vi "Build Array.vi"(8 "Msg ID":u16, 9 "Total no of Bytes":u16, 11 "Array":u8[](array[numeric])) -> (2 "Array Packets":u8[][](array[numeric]))   [LabVIEW 2020]
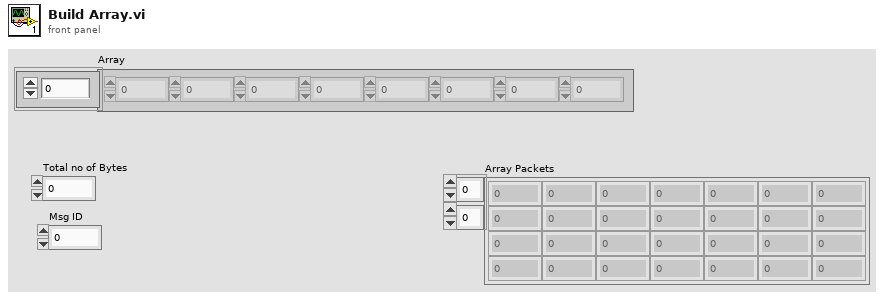
[diagram p1: front panel]
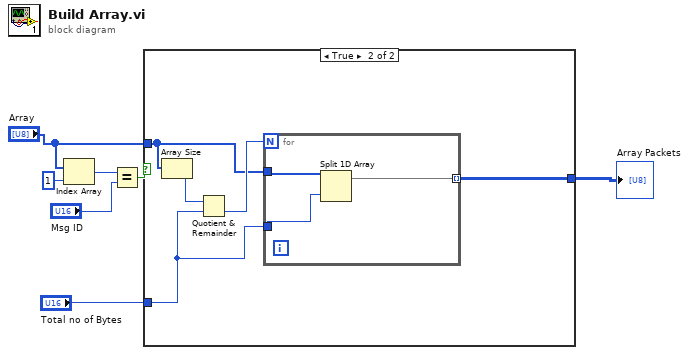
[diagram p0: block diagram]
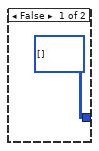
[diagram p2: hidden frame]
diagram:
  n1 = Index Array(array="Array", index=1) -> (element=w3:u8)
  n2 = Equal?(x=w3, y="Msg ID") -> (x = y?=w4:bool)
  n3 = case shown="True" w4 {
    tunnel: "Array" -> [_ w11]
    tunnel: "Total no of Bytes" -> [_ w10]
    tunnel: [u8[][] [] w9] -> w1
    frame False {
    }
    frame True {
      n4 = Array Size(array=w11) -> (size(s)=w13:i32)
      n5 = Quotient & Remainder(x=w13, y=w10) -> (floor(x/y)=w12:i32)  [unwired: 1 out]
      n6 = for {
        N: w12 -> [_]
        tunnel: w11 -> [w16]
        tunnel: w10 -> [w14]
        tunnel: [w15] -> w9 mode=indexing
        n7 = Split 1D Array(array=w16, index=w14) -> (first subarray=w15:u8[])  [unwired: 1 out]
      }
    }
  }
  "Array Packets" <- w1
